vi "Set Waveform to Constant.vi"(8 "Error In":errorcluster, 9 "Original Waveform":waveform(dbl), 10 "New Value":dbl) -> (0 "Error Out":errorcluster, 1 "New Waveform":waveform(dbl))   [LabVIEW 2021]
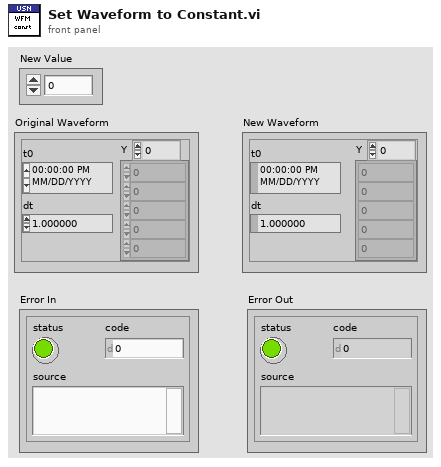
[diagram p1: front panel]
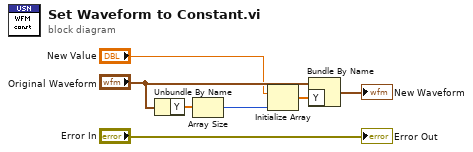
[diagram p0: block diagram]
diagram:
  n1 = Unbundle By Name("Original Waveform") -> ("Y"=w5:dbl[])
  n2 = Array Size(array=w5) -> (size(s)=w6:i32)
  n3 = Initialize Array("New Value", w6) -> (w7:dbl[])
  n4 = Bundle By Name(cluster="Original Waveform", "Y"=w7) -> (→"New Waveform":waveform(dbl))
  "Error Out" <- "Error In"
